vi "Window Title.vi"(0 "LV Doc in":refnum<class "LV Doc.lvclass">, 5 "VI Reference":refnum<vi>, 11 "error in (no error)":errorcluster) -> (4 "LV Doc out":refnum<class "LV Doc.lvclass">, 6 "Window Title":string, 15 "error out":errorcluster)   [LabVIEW 2016, in "LV Doc.lvclass"]
uses:
  LV Doc.lvclass
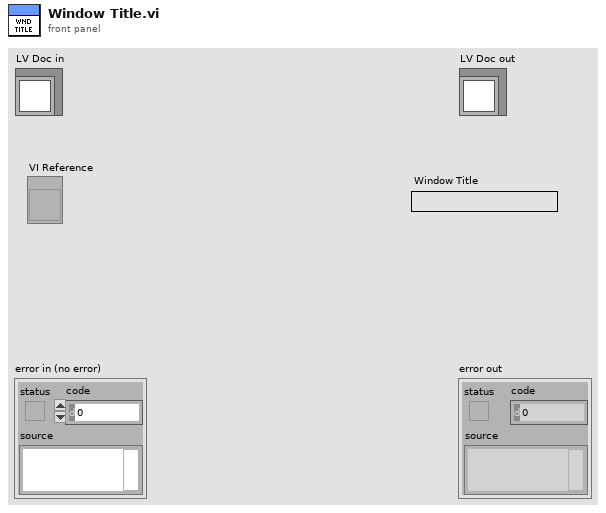
[diagram p1: front panel]
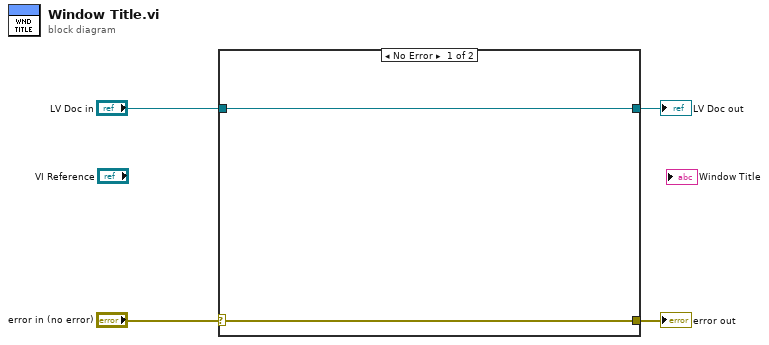
[diagram p0: block diagram]
diagram:
  n1 = case shown="No Error" "error in (no error)" {
    selector: "error in (no error)" -> [w5 w8]
    tunnel: [w5 w8] -> w3
    tunnel: [w6 w7] -> w1
    tunnel: "LV Doc in" -> [w6 w7]
    frame No Error {
    }
    frame Error {
    }
  }
  "error out" <- w3
  "LV Doc out" <- w1
